vi "MULTTCP_BlockConnsMgr.vi"(8 "error in (no error)":errorcluster, 9 "message back  queue":refnum<queue>, 10 "arg":string, 11 "action":enum16{"add", "delete", "find", "clear all"}(ring)) -> (0 "error out":errorcluster, 1 "found":bool, 2 "connection out":T1, 3 "send CB":bool)   [LabVIEW 2016]
uses:
  MULTTCP_BlockingStruct.ctl
panel:
  out "pending cb":T1[](array[typedef])
  in  "conn":T1
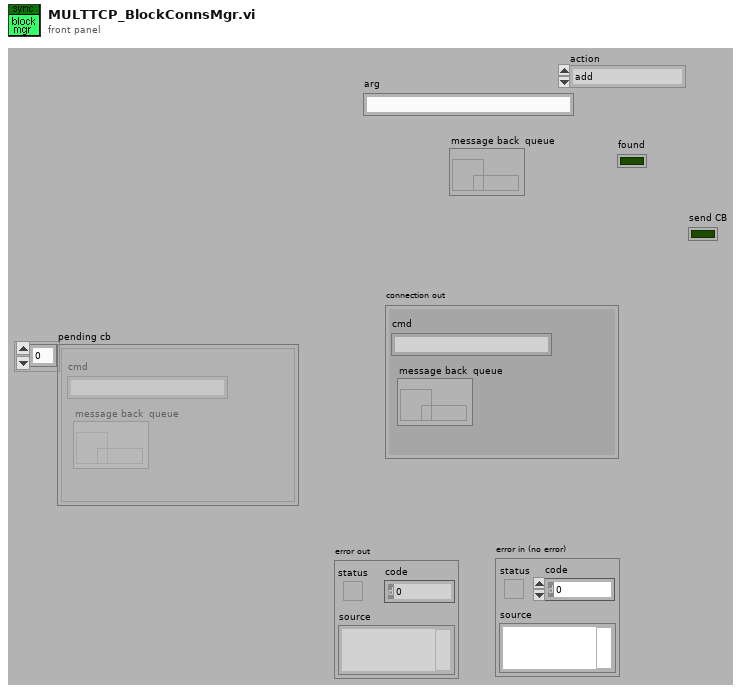
[diagram p1: front panel]
types:
  T1 = typedef "MULTTCP_BlockingStruct.ctl" = cluster{"cmd":string, "message back  queue":refnum<queue>}
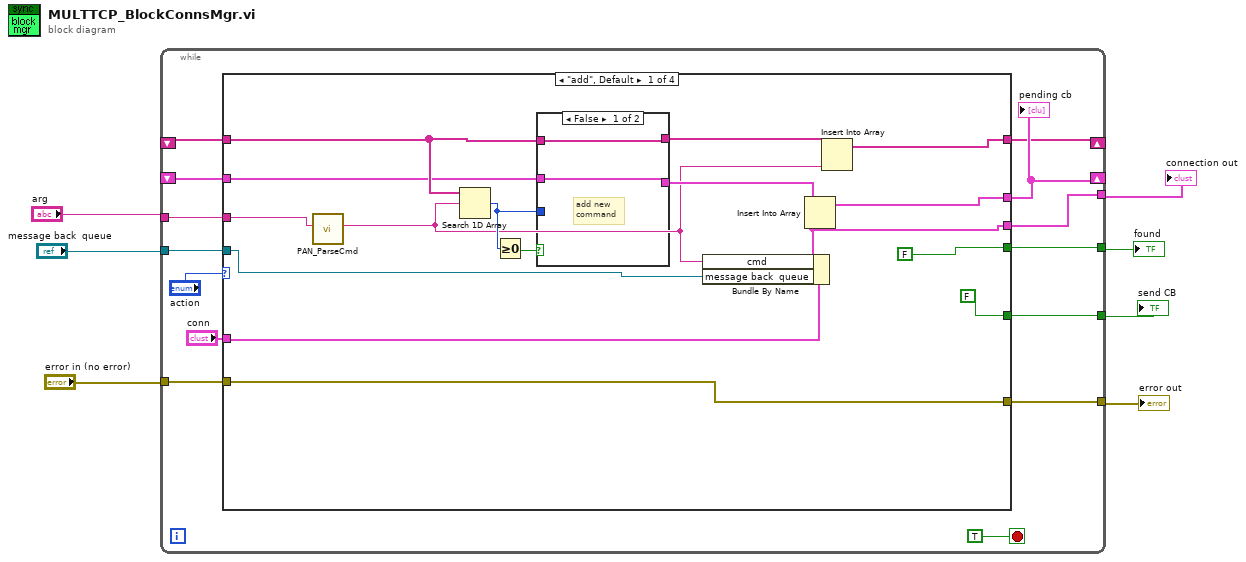
[diagram p0: block diagram]
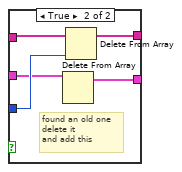
[diagram p2: hidden frame]
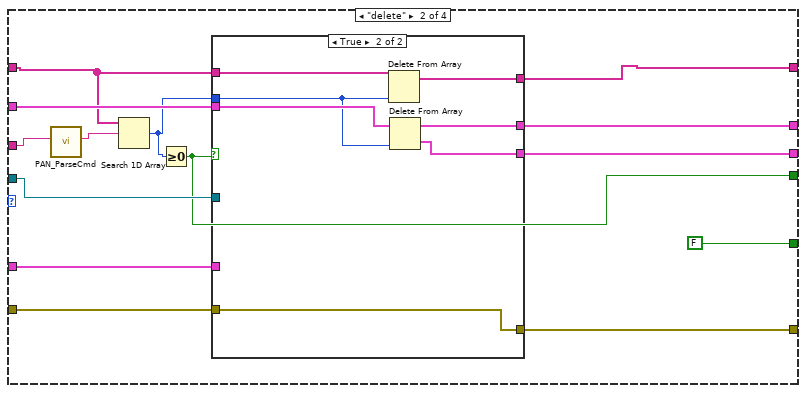
[diagram p3: hidden frame]
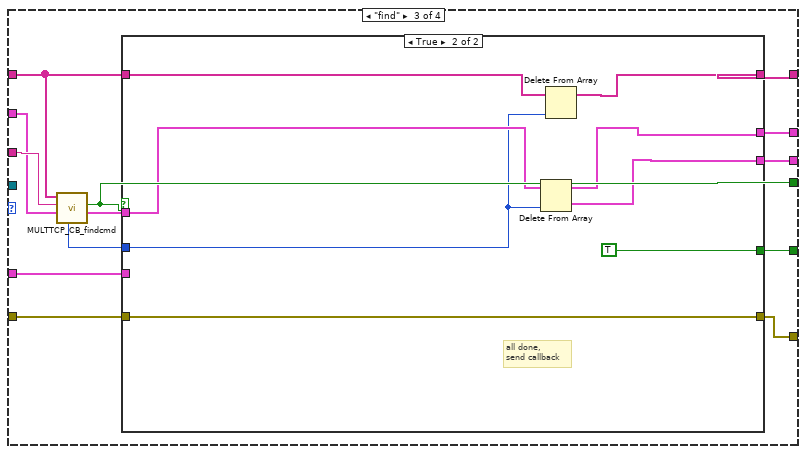
[diagram p5: hidden frame]
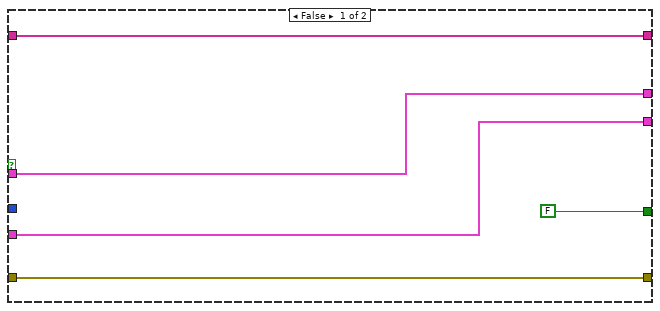
[diagram p6: hidden frame]
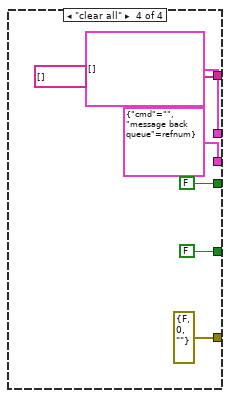
[diagram p7: hidden frame]
diagram:
  n1 = while {
    tunnel: "arg" -> [w19]
    tunnel: "message back  queue" -> [w18]
    shift-right: [w17] -> _
    shift-left: _ -> [w16]
    tunnel: "error in (no error)" -> [w15]
    tunnel: [w14] -> w4
    tunnel: [w13] -> w3
    tunnel: [w12] -> w2
    shift-right: [w9] -> _
    shift-left: _ -> [w10]
    tunnel: [w8] -> w1
    stop <- TRUE stop-if-true
    n2 = case shown="\"add\", Default" "action" {
      tunnel: w19 -> [w23 w46 w82 _]
      tunnel: w18 -> [w36 w56 _ _]
      tunnel: [w37 w58 w75 T1[] [] ("pending out")] -> w17
      tunnel: w16 -> [w26 w57 w81 _]
      tunnel: w15 -> [w35 w55 w79 _]
      tunnel: [w35 w54 w78 errorcluster {"status"=FALSE, "code"=0, "source"=""} ("error in (no error)")] -> w14
      tunnel: [FALSE ("status") w50 w72 FALSE ("found")] -> w13
      tunnel: [w33 w53 w74 T1 {"cmd"="", "message back  queue"=refnum} ("conn")] -> w12
      tunnel: "conn" -> [w32 w51 w73 _]
      tunnel: w10 -> [w28 w49 w77 _]
      tunnel: [w31 w48 w76 string[] []] -> w9
      tunnel: [FALSE FALSE w70 FALSE] -> w8
      frame "add", Default {
        n3 = call "PAN_ParseCmd.vi"("cmd in"=w23) -> ("cmd ref out"=w22:string)  [unwired: 10 out]
        n4 = Search 1D Array(1D array=w28, element=w22) -> (index of element=w27:i32)  [unwired: 1 out]
        n5 = Greater Or Equal To 0?(x=w27) -> (x >= 0?=w29:bool)
        n6 = case shown="False" w29 {
          tunnel: w28 -> [w39 w44]
          tunnel: w27 -> [_ w43]
          tunnel: w26 -> [w38 w42]
          tunnel: [w38 w41] -> w25
          tunnel: [w39 w40] -> w24
          frame False {
            # "add new\ncommand"
          }
          frame True {
            # "found an old one\ndelete it\nand add this"
            n7 = Delete From Array(array=w42) -> (array with subset deleted=w41:T1[])  [unwired: 2 in, 1 out]
            n8 = Delete From Array(array=w44, index=w43) -> (array with subset deleted=w40:string[])  [unwired: 1 in, 1 out]
          }
        }
        n9 = Bundle By Name(cluster=w32, "cmd"=w22, "message back  queue"=w36) -> (w33:T1)
        n10 = Insert Into Array(array=w25, new element=w33) -> (w37:T1[])  [unwired: 1 in]
        n11 = Insert Into Array(array=w24, new element=w22) -> (w31:string[])  [unwired: 1 in]
      }
      frame "delete" {
        n12 = call "PAN_ParseCmd.vi"("cmd in"=w46) -> ("cmd ref out"=w45:string)  [unwired: 10 out]
        n13 = Search 1D Array(1D array=w49, element=w45) -> (index of element=w52:i32)  [unwired: 1 out]
        n14 = Greater Or Equal To 0?(x=w52) -> (x >= 0?=w50:bool)
        n15 = case shown="True" w50 {
          tunnel: [w59 w69] -> w48
          tunnel: [w62 w68] -> w58
          tunnel: w57 -> [w62 w67]
          tunnel: w56 -> [_ _]
          tunnel: w55 -> [w60 w66]
          tunnel: [w60 w66] -> w54
          tunnel: [w61 w64] -> w53
          tunnel: w52 -> [_ w65]
          tunnel: w51 -> [w61 _]
          tunnel: w49 -> [w59 w63]
          frame False {
          }
          frame True {
            n16 = Delete From Array(array=w63, index=w65) -> (array with subset deleted=w69:string[])  [unwired: 1 in, 1 out]
            n17 = Delete From Array(array=w67, index=w65) -> (deleted portion=w64:T1, array with subset deleted=w68:T1[])  [unwired: 1 in]
          }
        }
      }
      frame "find" {
        n18 = call "MULTTCP_CB_findcmd.vi"("pending in"=w81, "message"=w82, "cmds"=w77) -> ("pending out"=w80:T1[], "found"=w72:bool, "cmd index"=w71:i32)  [unwired: 6 out]
        n19 = case shown="True" w72 {
          tunnel: w80 -> [w85 w92]
          tunnel: w79 -> [w87 w94]
          tunnel: [w87 w94] -> w78
          tunnel: w77 -> [w86 w95]
          tunnel: [w86 w93] -> w76
          tunnel: [w85 w91] -> w75
          tunnel: [w84 w90] -> w74
          tunnel: w73 -> [w84 _]
          tunnel: w71 -> [_ w89]
          tunnel: [FALSE TRUE] -> w70
          frame False {
          }
          frame True {
            # "all done,\nsend callback"
            n20 = Delete From Array(array=w92, index=w89) -> (deleted portion=w90:T1, array with subset deleted=w91:T1[])  [unwired: 1 in]
            n21 = Delete From Array(array=w95, index=w89) -> (array with subset deleted=w93:string[])  [unwired: 1 in, 1 out]
          }
        }
      }
      frame "clear all" {
      }
    }
    "pending cb" <- w17
  }
  "found" <- w3
  "error out" <- w4
  "connection out" <- w2
  "send CB" <- w1
